vi "Shutter Enum to binary.vi"(1 "Shutter to Open":T1=enum."Cy3 (532 nm)") -> (0 "Array":bool[](array[boolean]))   [LabVIEW 2018, in "Application.lvlib"]
uses:
  Application.lvlib
  Resources/Type Defs/Excitation.ctl
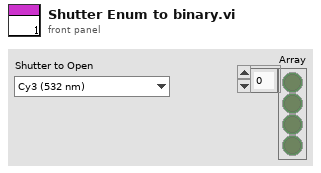
[diagram p1: front panel]
types:
  T1 = typedef "Excitation.ctl" = enum16{"Cy2 (473 nm)", "Cy3 (532 nm)", "Cy5 (639 nm)", "Cy7 (730 nm)", "Cy2/Cy3", "Cy3/Cy5", "Cy3/Cy7", "Cy5/Cy7"}
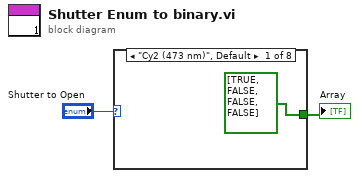
[diagram p0: block diagram]
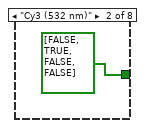
[diagram p2: hidden frame]
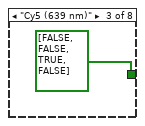
[diagram p3: hidden frame]
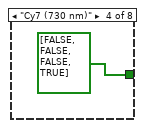
[diagram p4: hidden frame]
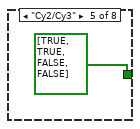
[diagram p5: hidden frame]
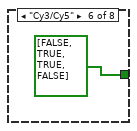
[diagram p6: hidden frame]
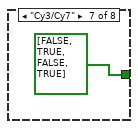
[diagram p7: hidden frame]
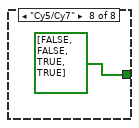
[diagram p8: hidden frame]
diagram:
  n1 = case shown="\"Cy2 (473 nm)\", Default" "Shutter to Open" {
    tunnel: [bool[] [TRUE, FALSE, FALSE, FALSE] bool[] [FALSE, TRUE, FALSE, FALSE] bool[] [FALSE, FALSE, TRUE, FALSE] bool[] [FALSE, FALSE, FALSE, TRUE] bool[] [TRUE, TRUE, FALSE, FALSE] bool[] [FALSE, TRUE, TRUE, FALSE] bool[] [FALSE, TRUE, FALSE, TRUE] bool[] [FALSE, FALSE, TRUE, TRUE]] -> w1
    frame "Cy2 (473 nm)", Default {
    }
    frame "Cy3 (532 nm)" {
    }
    frame "Cy5 (639 nm)" {
    }
    frame "Cy7 (730 nm)" {
    }
    frame "Cy2/Cy3" {
    }
    frame "Cy3/Cy5" {
    }
    frame "Cy3/Cy7" {
    }
    frame "Cy5/Cy7" {
    }
  }
  "Array" <- w1
